vi "receiver-8.6.vi"(6 "错误输入（无错误）":errorcluster, 7 "CAN端口":u8, 8 "设备索引号":u8, 9 "CAN卡类型":u8) -> (0 "错误输出":errorcluster, 1 "输出簇":T1, 2 "接收成功":bool, 3 "接收返回值":u32, 4 "VCI_Receive":T4 {"Rsv3" max=0 format="%x"; "Rsv2" min=101 format="%x"; "Rsv1" format="%x"; "Data8" format="%x"; "Data7" format="%x"; "Data6" format="%x"; "Data5" format="%x"; "Data4" format="%x"; "Data3" format="%x"; "Data2" format="%x"; "Data1" format="%x"; "DataLen" format="%x"; "ExternFlag" format="%x"; "RemoteFlag" format="%x"; "SendType" format="%x"; "TimeFlag" format="%x"; "TimeStamp" format="%x"; "ID" format="%x"}, 5 "VCI_CAN_OBJ_RN":T2(array[cluster])=[{"ID"=0, "TimeStamp"=0, "TimeFlag"=0, "SendType"=1, "RemoteFlag"=0, "ExternFlag"=0, "DataLen"=8, 0, 0, 0, 0, 0, 0, 0, 0, 0, 0, 0}, {"ID"=0, "TimeStamp"=0, "TimeFlag"=0, "SendType"=1, "RemoteFlag"=0, "ExternFlag"=0, "DataLen"=8, 0, 0, 0, 0, 0, 0, 0, 0, 0, 0, 0}, {"ID"=0, "TimeStamp"=0, "TimeFlag"=0, "SendType"=1, "RemoteFlag"=0, "ExternFlag"=0, "DataLen"=8, 0, 0, 0, 0, 0, 0, 0, 0, 0, 0, 0}, {"ID"=0, "TimeStamp"=0, "TimeFlag"=0, "SendType"=1, "RemoteFlag"=0, "ExternFlag"=0, "DataLen"=8, 0, 0, 0, 0, 0, 0, 0, 0, 0, 0, 0}, {"ID"=0, "TimeStamp"=0, "TimeFlag"=0, "SendType"=1, "RemoteFlag"=0, "ExternFlag"=0, "DataLen"=8, 0, 0, 0, 0, 0, 0, 0, 0, 0, 0, 0}, {"ID"=0, "TimeStamp"=0, "TimeFlag"=0, "SendType"=1, "RemoteFlag"=0, "ExternFlag"=0, "DataLen"=8, 0, 0, 0, 0, 0, 0, 0, 0, 0, 0, 0}, {"ID"=0, "TimeStamp"=0, "TimeFlag"=0, "SendType"=1, "RemoteFlag"=0, "ExternFlag"=0, "DataLen"=8, 0, 0, 0, 0, 0, 0, 0, 0, 0, 0, 0}, {"ID"=0, "TimeStamp"=0, "TimeFlag"=0, "SendType"=1, "RemoteFlag"=0, "ExternFlag"=0, "DataLen"=8, 0, 0, 0, 0, 0, 0, 0, 0, 0, 0, 0}, {"ID"=0, "TimeStamp"=0, "TimeFlag"=0, "SendType"=1, "RemoteFlag"=0, "ExternFlag"=0, "DataLen"=8, 0, 0, 0, 0, 0, 0, 0, 0, 0, 0, 0}, {"ID"=0, "TimeStamp"=0, "TimeFlag"=0, "SendType"=1, "RemoteFlag"=0, "ExternFlag"=0, "DataLen"=8, 0, 0, 0, 0, 0, 0, 0, 0, 0, 0, 0}])   [LabVIEW 2013]
uses:
  data/ControlCAN.dll
panel:
  out "数据":T3 {"ID" format="%x"}
  # "内部延时5ms"
  # "1245-------------------------------"
  # "接收成功"
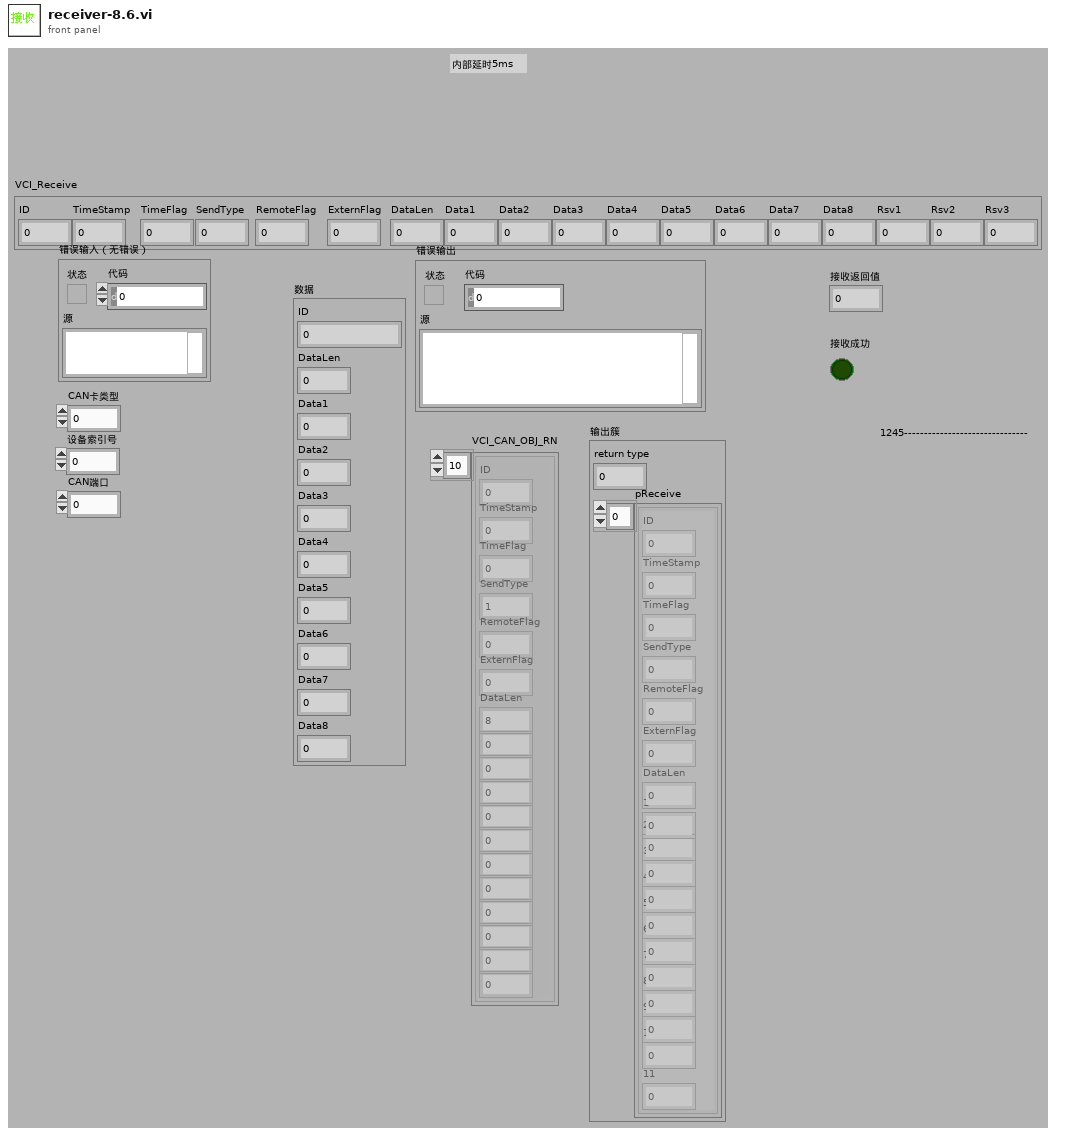
[diagram p1: front panel]
types:
  T1 = cluster{"return type":u32, "pReceive":cluster{"ID":u32, "TimeStamp":u32, "TimeFlag":u8, "SendType":u8, "RemoteFlag":u8, "ExternFlag":u8, "DataLen":u8, "1":u8, "2":u8, "3":u8, "4":u8, "5":u8, "6":u8, "7":u8, "8":u8, "9":u8, "10":u8, "11":u8}[]}
  T2 = cluster{"ID":u32, "TimeStamp":u32, "TimeFlag":u8, "SendType":u8, "RemoteFlag":u8, "ExternFlag":u8, "DataLen":u8, u8, u8, u8, u8, u8, u8, u8, u8, u8, u8, u8}[]
  T3 = cluster{"ID":u32, "DataLen":u8, "Data1":u8, "Data2":u8, "Data3":u8, "Data4":u8, "Data5":u8, "Data6":u8, "Data7":u8, "Data8":u8}
  T4 = cluster{"ID":u32, "TimeStamp":u32, "TimeFlag":u8, "SendType":u8, "RemoteFlag":u8, "ExternFlag":u8, "DataLen":u8, "Data1":u8, "Data2":u8, "Data3":u8, "Data4":u8, "Data5":u8, "Data6":u8, "Data7":u8, "Data8":u8, "Rsv1":u8, "Rsv2":u8, "Rsv3":u8}
  T5 = cluster{"return type":u32, "pReceive":cluster{"ID":u32, "TimeStamp":u32, "TimeFlag":u8, "SendType":u8, "RemoteFlag":u8, "ExternFlag":u8, "DataLen":u8, u8, u8, u8, u8, u8, u8, u8, u8, u8, u8, u8}[]}
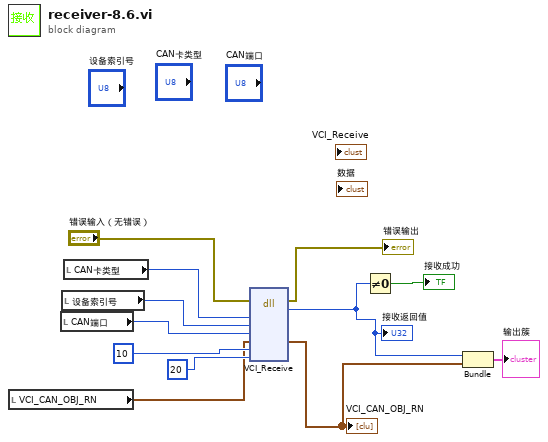
[diagram p0: block diagram]
diagram:
  n1 = local read "VCI_CAN_OBJ_RN"() -> (w4:T2)
  n2 = local read "CAN端口"() -> (w8:u8)
  n3 = local read "设备索引号"() -> (w9:u8)
  n4 = local read "CAN卡类型"() -> (w10:u8)
  n5 = dll-call lib="PTH1Fabs EDelan\t上位机BMS_Monitor - 91版_1dataControlCAN.dll" fn="VCI_Receive"(error in="错误输入（无错误）", "DeviceType"=w10, "DeviceInd"=w9, "CANInd"=w8, "pReceive"=w4, "Len"=10, "WaitTime"=20) -> (error out=→"错误输出":errorcluster, "return type"=w3:u32, "pReceive"=w2:T2)  [unwired: 7 in, 1 out]
  "接收返回值" <- w3
  "VCI_CAN_OBJ_RN" <- w2
  n6 = Not Equal To 0?(x=w3) -> (x != 0?=→"接收成功":bool)
  n7 = Bundle("return type"=w3, "pReceive"=w2) -> (→"输出簇":T5)  [unwired: 1 in]
